vi "To MCP Name.vi"(11 "unformatted name":string) -> (3 "MCP name":string)   [LabVIEW 2025, in "MCP Server.lvlib"]
doc: "removes spaces and moves to lower case to comply with MCP naming conventions for tool names, prompt names etc."
uses:
  MCP Server.lvlib
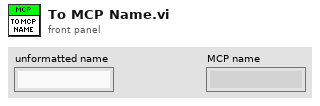
[diagram p1: front panel]
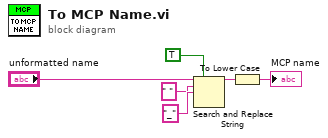
[diagram p0: block diagram]
diagram:
  n1 = Search and Replace String(replace all?=TRUE ("replace all? (F)"), input string="unformatted name", search string=" ", replace string="_" ("replace string (\"\")")) -> (result string=w3:string)  [unwired: 4 in, 3 out]
  n2 = To Lower Case(string=w3) -> (all lower case string=→"MCP name":string)
